vi "graphs.vi"() -> ()   [LabVIEW 2020]
panel:
  out "XY Graph":cluster{i32[], dbl[]}(graph)
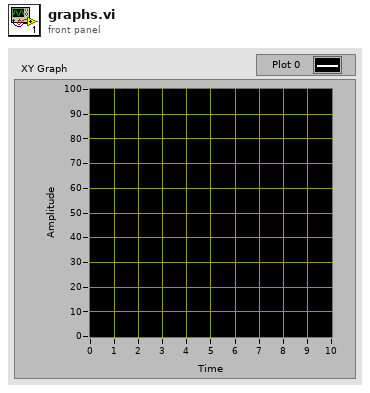
[diagram p1: front panel]
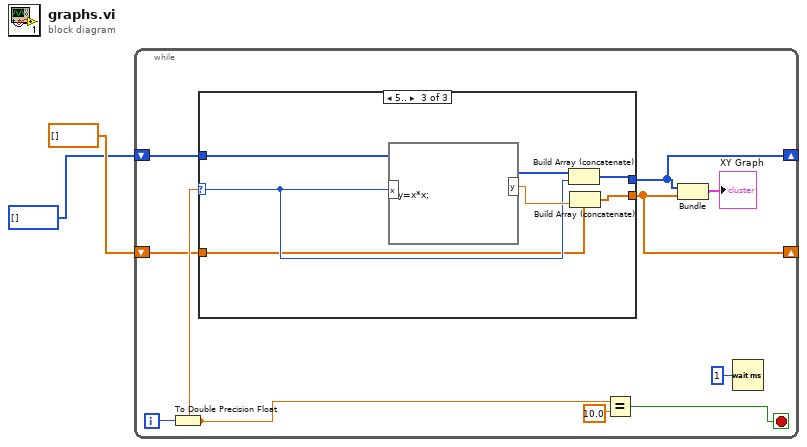
[diagram p0: block diagram]
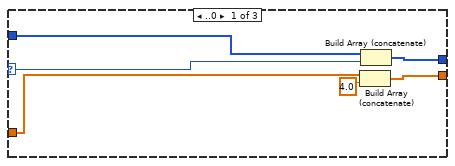
[diagram p2: hidden frame]
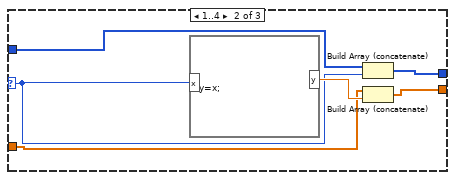
[diagram p3: hidden frame]
diagram:
  n1 = while {
    shift-right: [w5] -> _
    shift-left: dbl[] [] -> [w6]
    shift-right: [w3] -> _
    shift-left: i32[] [] -> [w4]
    i -> [w8]
    stop <- w10 stop-if-true
    n2 = To Double Precision Float(number=w8) -> (double precision float=w9:dbl)
    n3 = case shown="5.." w9 {
      selector: w9 -> [w15 w21 w27]
      tunnel: [w17 w23 w29] -> w5
      tunnel: [w16 w24 w28] -> w3
      tunnel: w6 -> [w14 w19 w26]
      tunnel: w4 -> [w13 w20 w25]
      frame ..0 {
        n4 = Build Array (concatenate)(w14, 4.0) -> (w17:dbl[])
        n5 = Build Array (concatenate)(w13, w15) -> (w16:i32[])
      }
      frame 1..4 {
        n6 = formula code="y=x;"("x"=w21) -> ("y"=w22:dbl)
        n7 = Build Array (concatenate)(w20, w21) -> (w24:i32[])
        n8 = Build Array (concatenate)(w19, w22) -> (w23:dbl[])
      }
      frame 5.. {
        n9 = formula code="y=x*x;"("x"=w27) -> ("y"=w30:dbl)
        n10 = Build Array (concatenate)(w25, w27) -> (w28:i32[])
        n11 = Build Array (concatenate)(w26, w30) -> (w29:dbl[])
      }
    }
    n12 = Equal?(x=w9, y=10.0) -> (x = y?=w10:bool)
    n13 = Bundle(w3, w5) -> (→"XY Graph":cluster{i32[], dbl[]})  [unwired: 1 in]
    n14 = Wait (ms)(milliseconds to wait=u32 1) -> ()  [unwired: 1 out]
  }
